vi "Periferal Measurement Saver.vi"(0 "Experiment Index":dynamicdata(waveform), 1 "Session Index":dynamicdata(waveform), 2 "Dynamic Data":dynamicdata(waveform), 3 "Feature Index":dynamicdata(waveform), 4 "Frequency Saver?":bool=TRUE) -> ()   [LabVIEW 2023]
uses:
  <vilib>/express/express shared/transition.llb/Dynamic To Waveform Array.vi
  <vilib>/express/express signal manip/GetorSetDDTAttributes/Set DDT Attributes/SetT0.vi
  <vilib>/express/express shared/transition.llb/Waveform Array To Dynamic.vi
  <vilib>/express/express signal manip/GetorSetDDTAttributes/Set DDT Attributes/Set DDT Properties.xnode
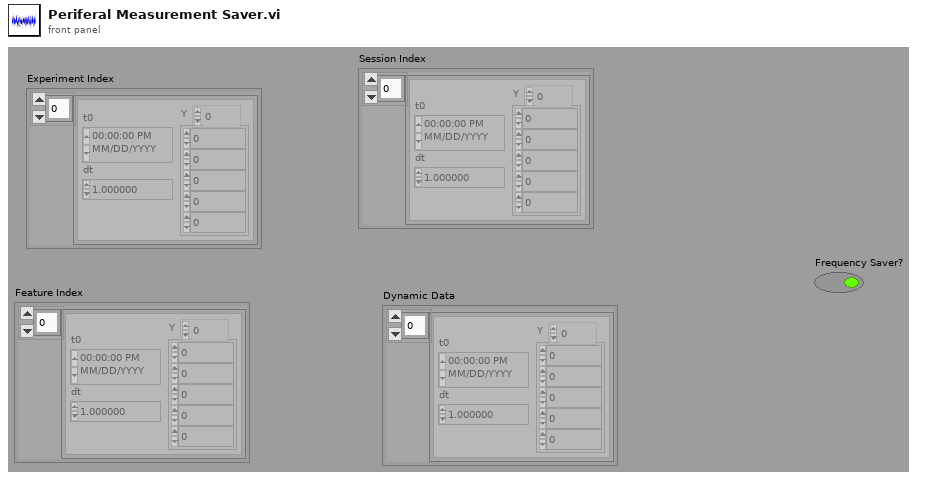
[diagram p1: front panel]
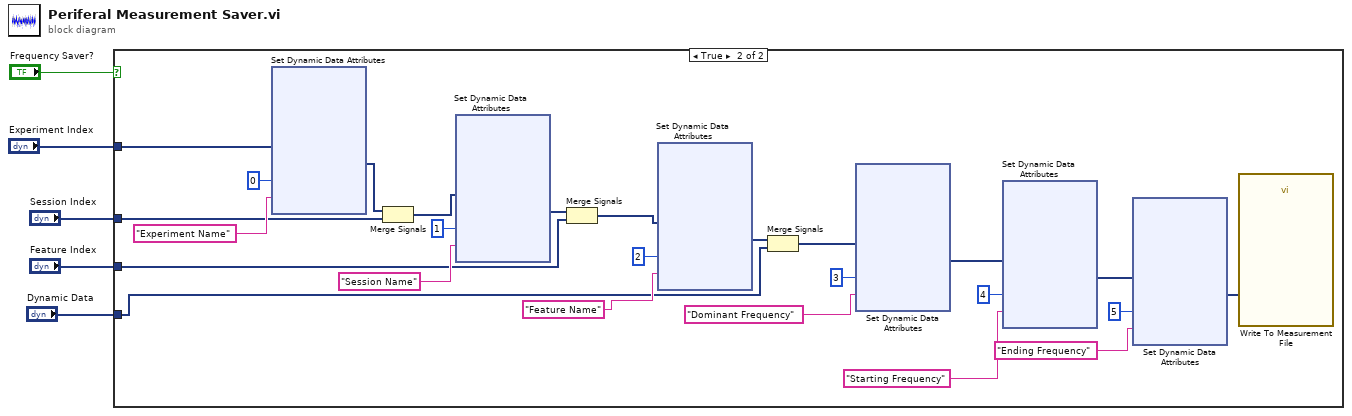
[diagram p0: block diagram]
diagram:
  n1 = case shown="True" "Frequency Saver?" {
    tunnel: "Dynamic Data" -> [_ w6]
    tunnel: "Experiment Index" -> [_ w16]
    tunnel: "Session Index" -> [_ w15]
    tunnel: "Feature Index" -> [_ w7]
    frame False {
    }
    frame True {
      n2 = xnode "Set Dynamic Data Attributes"("Signals In"=w16, "Signal Index"=0, "Signal Name"="Experiment Name") -> ("Signals Out"=w14:dynamicdata)  [unwired: 1 in, 1 out]
      n3 = Merge Signals(w14, w15) -> (w13:dynamicdata)
      n4 = xnode "Set Dynamic Data Attributes"("Signals In"=w13, "Signal Index"=1, "Signal Name"="Session Name") -> ("Signals Out"=w8:dynamicdata)  [unwired: 1 in, 1 out]
      n5 = Merge Signals(w8, w7) -> (w9:dynamicdata)
      n6 = xnode "Set Dynamic Data Attributes"("Signals In"=w9, "Signal Index"=2, "Signal Name"="Feature Name") -> ("Signals Out"=w12:dynamicdata)  [unwired: 1 in, 1 out]
      n7 = Merge Signals(w12, w6) -> (w17:dynamicdata)
      n8 = xnode "Set Dynamic Data Attributes"("Signals In"=w17, "Signal Index"=3, "Signal Name"="Dominant Frequency") -> ("Signals Out"=w29:dynamicdata)  [unwired: 1 in, 1 out]
      n9 = xnode "Set Dynamic Data Attributes"("Signals In"=w29, "Signal Index"=4, "Signal Name"="Starting Frequency") -> ("Signals Out"=w24:dynamicdata)  [unwired: 1 in, 1 out]
      n10 = xnode "Set Dynamic Data Attributes"("Signals In"=w24, "Signal Index"=5, "Signal Name"="Ending Frequency") -> ("Signals Out"=w22:dynamicdata)  [unwired: 1 in, 1 out]
      n11 = call "Write To Measurement File"("Signals"=w22) -> ()  [unwired: 16 in, 3 out]
    }
  }
